vi "MIDI Controller.vi"() -> ()   [LabVIEW 2017]
panel:
  out "CTAH Direct":sgl
  out "TCHX Direct":sgl
  out "Pump Direct":sgl
  out "Power Out":sgl
  out "MIDI Preview":T1
  in  "Activation":bool
  in  "stop":bool
  out "MIDI Connected":bool
  # "MIDI Output"
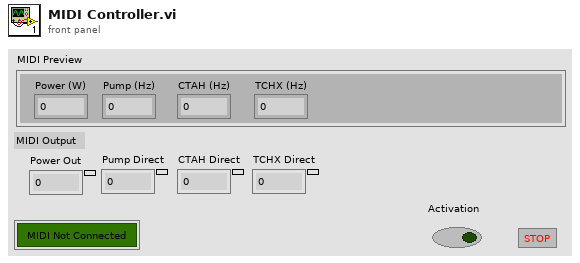
[diagram p1: front panel]
types:
  T1 = cluster{"Power (W)":dbl, "Pump (Hz)":dbl, "CTAH (Hz)":dbl, "TCHX (Hz)":dbl}
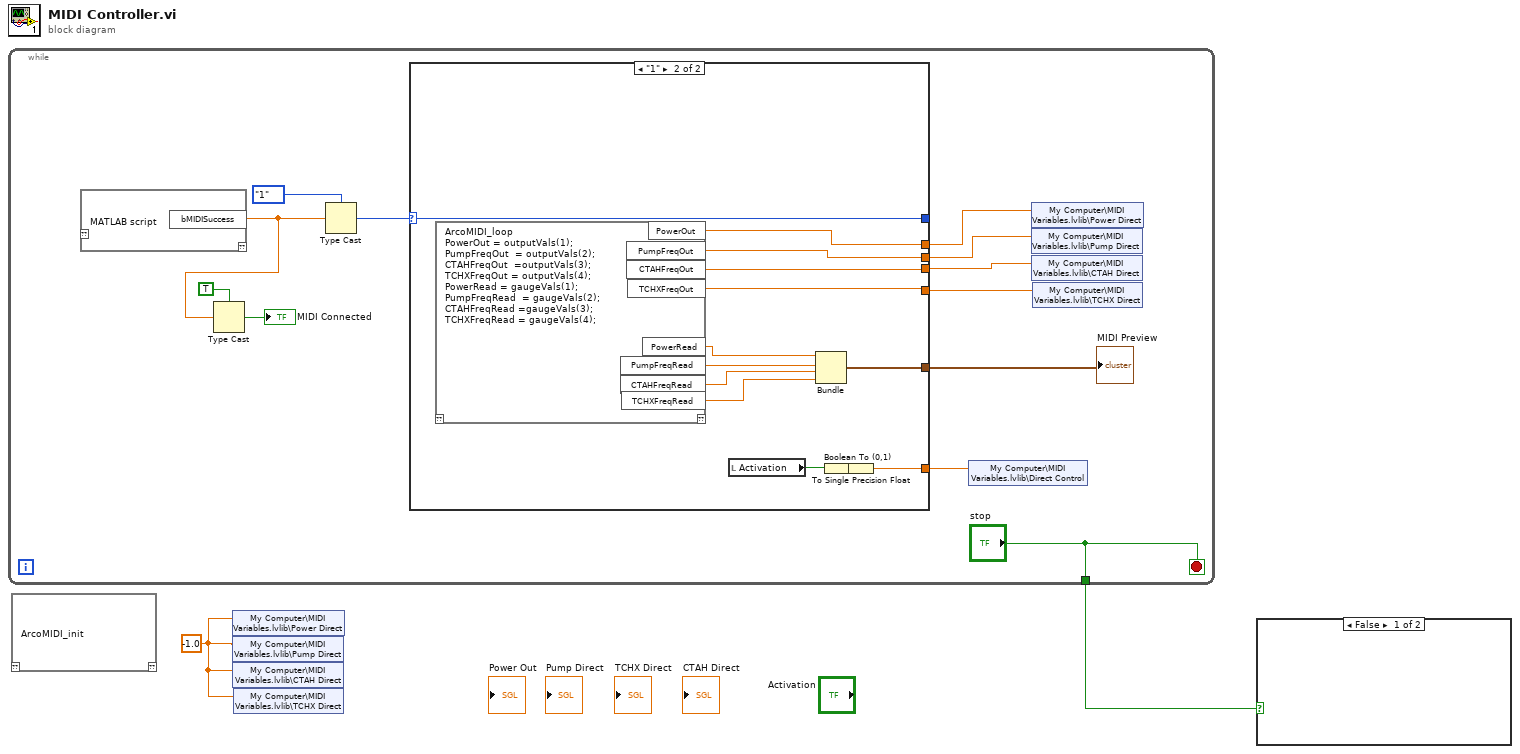
[diagram p0: block diagram]
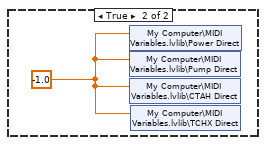
[diagram p2: hidden frame]
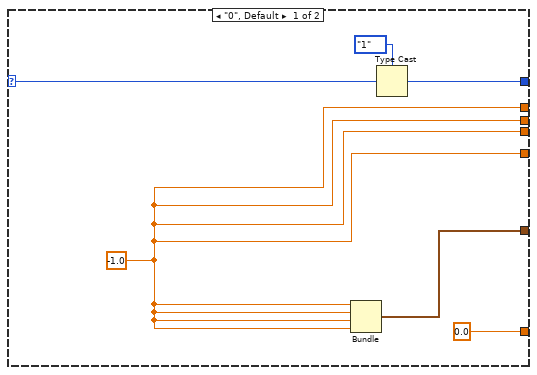
[diagram p3: hidden frame]
diagram:
  w1 = -1.0
  n1 = while {
    tunnel: ["stop"] -> w2
    stop <- "stop" stop-if-true
    n2 = script code="MATLAB script"() -> ("bMIDISuccess"=w10:dbl)  [unwired: 1 in, 1 out]
    n3 = Type Cast(type=TRUE, x=w10) -> (*(type *) &x=→"MIDI Connected":bool)
    n4 = Type Cast(type=enum16{"0", "1"}."1", x=w10) -> (*(type *) &x=w13:enum16{"0", "1"})
    n5 = case shown="\"1\"" w13 {
      selector: w13 -> [w18 w33]
      tunnel: [w19 w33] -> _
      tunnel: [w17 w28] -> w8
      tunnel: [w15 w27] -> w7
      tunnel: [w15 w26] -> w6
      tunnel: [w15 w25] -> w5
      tunnel: [w15 w24] -> w4
      tunnel: [0.0 w21] -> w3
      frame "0", Default {
        w15 = -1.0
        n6 = Bundle(w15, w15, w15, w15) -> (w17:cluster{dbl, dbl, dbl, dbl})  [unwired: 1 in]
        n7 = Type Cast(type=enum16{"0", "1"}."1", x=w18) -> (*(type *) &x=w19:enum16{"0", "1"})
      }
      frame "1" {
        n8 = script code="ArcoMIDI_loop\nPowerOut = outputVals(1);\nPumpFreqOut  = outputVals(2);\nCTAHFreqOut  =outputVals(3);\nTCHXFreqOut = outputVals(4);\nPowerRead = gaugeVals(1);\nPumpFreqRead  = gaugeVals(2);\nCTAHFreqRead =gaugeVals(3);\nTCHXFreqRead = gaugeVals(4);"() -> ("PowerOut"=w27:dbl, "PumpFreqOut"=w26:dbl, "CTAHFreqOut"=w25:dbl, "TCHXFreqOut"=w24:dbl, "PowerRead"=w32:dbl, "PumpFreqRead"=w31:dbl, "CTAHFreqRead"=w30:dbl, "TCHXFreqRead"=w29:dbl)  [unwired: 1 in, 1 out]
        n9 = local read "Activation"() -> (w23:bool)
        n10 = Bundle(w32, w31, w30, w29) -> (w28:cluster{dbl, dbl, dbl, dbl})  [unwired: 1 in]
        n11 = Boolean To (0,1)(Boolean=w23) -> (0, 1=w22:i16)
        n12 = To Single Precision Float(number=w22) -> (single precision float=w21:sgl)
      }
    }
    "MIDI Preview" <- w8
    n13 = shared-variable "My Computer\\MIDI Variables.lvlib\\Direct Control"(w3) -> ()  [unwired: 1 in, 1 out]
    n14 = shared-variable "My Computer\\MIDI Variables.lvlib\\Power Direct"(w7) -> ()  [unwired: 1 in, 1 out]
    n15 = shared-variable "My Computer\\MIDI Variables.lvlib\\Pump Direct"(w6) -> ()  [unwired: 1 in, 1 out]
    n16 = shared-variable "My Computer\\MIDI Variables.lvlib\\CTAH Direct"(w5) -> ()  [unwired: 1 in, 1 out]
    n17 = shared-variable "My Computer\\MIDI Variables.lvlib\\TCHX Direct"(w4) -> ()  [unwired: 1 in, 1 out]
  }
  n18 = script code="ArcoMIDI_init"() -> ()  [unwired: 1 in, 1 out]
  n19 = shared-variable "My Computer\\MIDI Variables.lvlib\\Power Direct"(w1) -> ()  [unwired: 1 in, 1 out]
  n20 = shared-variable "My Computer\\MIDI Variables.lvlib\\Pump Direct"(w1) -> ()  [unwired: 1 in, 1 out]
  n21 = shared-variable "My Computer\\MIDI Variables.lvlib\\CTAH Direct"(w1) -> ()  [unwired: 1 in, 1 out]
  n22 = shared-variable "My Computer\\MIDI Variables.lvlib\\TCHX Direct"(w1) -> ()  [unwired: 1 in, 1 out]
  n23 = case shown="False" w2 {
    frame False {
    }
    frame True {
      w34 = -1.0
      n24 = shared-variable "My Computer\\MIDI Variables.lvlib\\Power Direct"(w34) -> ()  [unwired: 1 in, 1 out]
      n25 = shared-variable "My Computer\\MIDI Variables.lvlib\\Pump Direct"(w34) -> ()  [unwired: 1 in, 1 out]
      n26 = shared-variable "My Computer\\MIDI Variables.lvlib\\CTAH Direct"(w34) -> ()  [unwired: 1 in, 1 out]
      n27 = shared-variable "My Computer\\MIDI Variables.lvlib\\TCHX Direct"(w34) -> ()  [unwired: 1 in, 1 out]
    }
  }
